vi "HFRR ADV v024 new software.vi"() -> ()   [LabVIEW 2025] (continued)
            n792 = call "IMAGE PATH CREATION PY.vi"("error in (no error)"=w991, "File Name :"=w992) -> ("error out"=w990:errorcluster, "File Path"=w978:path, "File Path String:"=w973:string)  [unwired: 7 in]
            n793 = Match Pattern(string=w986, regular expression=",") -> (before substring=w972:string)  [unwired: 1 in, 3 out]
            n794 = local read "Calibration Tab"() -> (w975:enum32{"Measrument", "Calibrate"})
            n795 = call "Stall Data Flow.vim"("value in"=w990, "milliseconds to wait"=u32 250) -> ("value out"=w974:errorcluster)  [unwired: 1 out]
            n796 = Equal?(x=w972, y="\"rectangle\"") -> (x = y?=w983:bool)
            n797 = case shown="False" w983 {
              tunnel: w982 -> [w1037 w1092]
              tunnel: w979 -> [_ w1083]
              tunnel: cluster{"major":dbl, "minor":dbl, "average":dbl} {"major"=0.0, "minor"=0.0, "average"=0.0} -> [w1035 w1079]
              tunnel: [w1034 w1076] -> w977
              tunnel: w972 -> [w1036 _]
              tunnel: w979 -> [w1033 _]
              frame False {
                n798 = Equal?(x=w1036, y="\"line\"") -> (x = y?=w1038:bool)
                n799 = case shown="True" w1038 {
                  tunnel: w1037 -> [_ w1053]
                  tunnel: w1035 -> [w1040 w1052]
                  tunnel: [w1040 w1050] -> w1034
                  tunnel: w1033 -> [_ w1049]
                  frame False {
                  }
                  frame True {
                    w1048 = 0.0 ("Major Axis")
                    n800 = Match Pattern(string=w1053, regular expression="\"length_px\":") -> (after substring=w1051:string)  [unwired: 1 in, 3 out]
                    n801 = property on="Major Axis" class="DigNum (strict)"("Caption.Text"="") -> ()  [unwired: 2 in, 2 out]
                    n802 = property on="Minor Axis" class="DigNum (strict)"("Caption.Text"="") -> ()  [unwired: 2 in, 2 out]
                    n803 = property on="Average" class="DigNum (strict)"("Caption.Text"="Line") -> ()  [unwired: 2 in, 2 out]
                    n804 = Fract/Exp String To Number(string=w1051, default (0 dbl)=0.0 ("default (0 DBL)")) -> (number=w1047:dbl)  [unwired: 2 in, 1 out]
                    "Pixel Value" <- w1047
                    n805 = Multiply(x=w1047, y=w1049) -> (x*y=w1060:dbl)
                    n806 = Multiply(x=w1060, y=1000.0) -> (x*y=w1043:dbl)
                    n807 = Divide(x=w1043, y=1000.0) -> (x/y=w1046:dbl)
                    n808 = local write "Measurment (mm)"(w1046) -> ()
                    n809 = Bundle By Name(cluster=w1052, "average"=w1043) -> (w1050:cluster{"major":dbl, "minor":dbl, "average":dbl})
                    n810 = Number To Fractional String(number=w1043, precision (6)=i16 1) -> (F-format string=w1042:string)  [unwired: 2 in]
                    n811 = local write "Minor Axis"(w1048) -> ()
                    n812 = local write "Major Axis"(w1048) -> ()
                    n813 = Fract/Exp String To Number(string=w1042) -> (number=w1041:dbl)  [unwired: 3 in, 1 out]
                    n814 = local write "Average"(w1041) -> ()
                  }
                }
              }
              frame True {
                w1080 = 1000.0 ("y")
                w1086 = 0.0 ("default (0 DBL)")
                n815 = Match Pattern(string=w1092, regular expression=" \"width_px\":") -> (after substring=w1090:string)  [unwired: 1 in, 3 out]
                n816 = Match Pattern(string=w1090, regular expression="\"height_px\":") -> (before substring=w1088:string, after substring=w1087:string)  [unwired: 1 in, 2 out]
                n817 = Fract/Exp String To Number(string=w1088, default (0 dbl)=w1086) -> (number=w1085:dbl)  [unwired: 2 in, 1 out]
                n818 = Fract/Exp String To Number(string=w1087, default (0 dbl)=w1086) -> (number=w1084:dbl)  [unwired: 2 in, 1 out]
                n819 = Multiply(x=w1085, y=w1083) -> (x*y=w1082:dbl)
                n820 = Multiply(x=w1084, y=w1083) -> (x*y=w1081:dbl)
                n821 = Multiply(x=w1082, y=w1080) -> (x*y=w1066:dbl)
                n822 = Multiply(x=w1081, y=w1080) -> (x*y=w1064:dbl)
                n823 = Add(x=w1066, y=w1064) -> (x+y=w1078:dbl)
                n824 = property on="Major Axis" class="DigNum (strict)"("Caption.Text"="Major Axis") -> ()  [unwired: 2 in, 2 out]
                n825 = property on="Minor Axis" class="DigNum (strict)"("Caption.Text"="Minor Axis") -> ()  [unwired: 2 in, 2 out]
                n826 = property on="Average" class="DigNum (strict)"("Caption.Text"="Average") -> ()  [unwired: 2 in, 2 out]
                n827 = Divide(x=w1078, y=2.0) -> (x/y=w1062:dbl)
                n828 = Bundle By Name(cluster=w1079, "major"=w1066, "minor"=w1064, "average"=w1062) -> (w1076:cluster{"major":dbl, "minor":dbl, "average":dbl})
                n829 = Number To Fractional String(number=w1064, precision (6)=i16 1) -> (F-format string=w1071:string)  [unwired: 2 in]
                n830 = Number To Fractional String(number=w1062, precision (6)=i16 1) -> (F-format string=w1072:string)  [unwired: 2 in]
                n831 = Number To Fractional String(number=w1066, precision (6)=i16 1) -> (F-format string=w1070:string)  [unwired: 2 in]
                n832 = Fract/Exp String To Number(string=w1071) -> (number=w1063:dbl)  [unwired: 3 in, 1 out]
                n833 = Fract/Exp String To Number(string=w1072) -> (number=w1061:dbl)  [unwired: 3 in, 1 out]
                n834 = Fract/Exp String To Number(string=w1070) -> (number=w1065:dbl)  [unwired: 3 in, 1 out]
                n835 = local write "Major Axis"(w1065) -> ()
                n836 = local write "Average"(w1061) -> ()
                n837 = local write "Minor Axis"(w1063) -> ()
              }
            }
            n838 = case shown="\"Measrument\", Default" w975 {
              tunnel: w978 -> [w1005 _]
              tunnel: w977 -> [w1004 _]
              tunnel: [w1001 w1030] -> w976
              tunnel: w974 -> [w1003 w1030]
              tunnel: w973 -> [w1002 _]
              tunnel: w970 -> [w1000 _]
              frame "Measrument", Default {
                n839 = stacked-sequence {
                  tunnel: w1005 -> [w1023 _]
                  tunnel: w1004 -> [w1021 _]
                  tunnel: w1003 -> [w1019 _]
                  tunnel: w1002 -> [w1018 _]
                  tunnel: [w1013 _] -> w1001
                  tunnel: w1000 -> [w1006 _]
                  frame #0 {
                    n840 = call "IMAGE ANALYSIS.vi"("Enum"=POST_ANALYSIS_ENUM."SAVE IMAGE", "error in"=w1019, "IMAGE FILE PATH"=w1018) -> ("error out"=w1017:errorcluster)  [unwired: 7 in, 1 out]
                    n841 = call "Stall Data Flow.vim"("value in"=w1017, "milliseconds to wait"=u32 1000) -> ("value out"=w1008:errorcluster)  [unwired: 1 out]
                    n842 = local read "Test File List :"() -> (w1025:string)
                    n843 = call "IMAGE ANALYSIS.vi"("Enum"=POST_ANALYSIS_ENUM."MINIMIZE UI", "error in"=w1008) -> ("error out"=w1015:errorcluster)  [unwired: 8 in, 1 out]
                    n844 = Bundle By Name(cluster=T25 {"File Name"="", "Test Method"="", "Operator"="", "Fuel Description"="", "Date and time"=""} ("Main Ref"), "Test Method"=w1006, "File Name"=w1025) -> (w1026:T25)
                    n845 = call "Stall Data Flow.vim"("value in"=w1015, "milliseconds to wait"=u32 1500) -> ("value out"=w1010:errorcluster)  [unwired: 1 out]
                    n846 = call "duf file read.vi"("error in (no error)"=w1010, "Main Ref"=w1026) -> ("error out"=w1024:errorcluster, "Main Ref 2"=w1022:T25)  [unwired: 8 in]
                    n847 = call "DETECTION REPORT for manual.vi"("error in (no error)"=w1024, "return value 3"=w1021, "Image File Path"=w1023, "Main Ref"=w1022) -> ("error out"=w1020:errorcluster)  [unwired: 7 in]
                    n848 = call <vilib>:"Clear Errors.vi"("error in (no error)"=w1020) -> ("error out"=w1011:errorcluster)  [unwired: 5 in, 1 out]
                    n849 = call "IMAGE ANALYSIS.vi"("Enum"=POST_ANALYSIS_ENUM."MINIMIZE UI", "error in"=w1011) -> ("error out"=w1013:errorcluster)  [unwired: 8 in, 1 out]
                  }
                  frame #1 {
                    n850 = local write "Main Tab"(T2."HOME" ("Main Tab")) -> ()
                    n851 = local write "Main Dashboard Buttons"(T1."Home" ("Main Dashboard Buttons")) -> ()
                  }
                }
              }
              frame "Calibrate" {
              }
            }
          }
          frame #2 {
            n852 = Not(x=w1095) -> (.not. x?=w1094:bool)
            n853 = local write "Confirm Measrurement"(w1094) -> ()
            n854 = local read "Calibration Tab"() -> (w1093:enum32{"Measrument", "Calibrate"})
            n855 = case shown="\"Measrument\", Default" w1093 {
              frame "Measrument", Default {
                (unwired) T20."HOME" ("Main Tab")
                n856 = local write "Main Tab"(T2."HOME" ("Main Tab")) -> ()
              }
              frame "Calibrate" {
              }
            }
          }
        }
      }
    }
    n857 = local read "Humidity"() -> (w838:bool)
    n858 = local read "Save Change"() -> (w843:bool)
    n859 = local read "Calibrate"() -> (w844:bool)
    n860 = local read "Auto Start Test"() -> (w839:bool)
    n861 = case shown="True" w844 {
      selector: w844 -> [_ w951]
      frame False {
      }
      frame True {
        n862 = Not(x=w951) -> (.not. x?=w950:bool)
        n863 = local write "Calibrate"(w950) -> ()
        n864 = local write "Calibration Tab"(enum32{"Measrument", "Calibrate"}."Calibrate" ("Calibration Tab")) -> ()
      }
    }
    n865 = case shown="True" w843 {
      selector: w843 -> [_ w895]
      frame False {
      }
      frame True {
        n866 = stacked-sequence {
          tunnel: w895 -> [_ _ _ _ w949]
          frame #0 {
            n867 = call "IMAGE ANALYSIS.vi"("Enum"=POST_ANALYSIS_ENUM."HIDE UI") -> ()  [unwired: 9 in, 2 out]
          }
          frame #1 {
            n868 = local read "100x gain"() -> (w897:dbl)
            n869 = local read "10x Gain"() -> (w898:dbl)
            n870 = local read "5x Gain"() -> (w899:dbl)
            n871 = Number To Fractional String(number=w898, width (-)=i16 4, precision (6)=i16 7) -> (F-format string=w920:string)  [unwired: 1 in]
            n872 = Number To Fractional String(number=0.0, width (-)=i16 4, precision (6)=i16 7) -> (F-format string=w915:string)  [unwired: 1 in]
            n873 = Number To Fractional String(number=w897, width (-)=i16 4, precision (6)=i16 7) -> (F-format string=w903:string)  [unwired: 1 in]
            n874 = Number To Fractional String(number=w899, width (-)=i16 10 ("precision (6)"), precision (6)=i16 7) -> (F-format string=w929:string)  [unwired: 1 in]
            n875 = Concatenate Strings("[CH1]" ("string"), w929, " - 5x Gain" ("string"), "\r") -> (w919:string)
            n876 = Concatenate Strings("[CH2]" ("string"), w920, " - 10x Gain" ("string"), "\r") -> (w918:string)
            n877 = Concatenate Strings("[CH3]" ("string"), w915, " - 20x Gain" ("string"), "\r") -> (w909:string)
            n878 = Concatenate Strings("[CH4]" ("string"), w903, " - 100x Gain" ("string"), "\r") -> (w902:string)
            n879 = String To Path(string="C:\\LAB-IQ\\Image Calibrate v01.dcf") -> (path=w932:path)
            n880 = Concatenate Strings(w919, w918, w909, w902) -> (w917:string)
            n881 = call <vilib>:"Write Characters To File.vi"("append to file? (new file:F)"=FALSE, "character string"=w917, "file path (dialog if empty)"=w932) -> ()  [unwired: 2 in, 1 out]
          }
          frame #2 {
            n882 = String To Path(string="C:\\LAB-IQ\\Image Calibrate v01.dcf") -> (path=w935:path)
            n883 = Open/Create/Replace File ("Open File")(file path (use dialog)=w935) -> (refnum out=w936:refnum<file>)  [unwired: 5 in, 2 out]
            n884 = for {
              N: 4 -> [_]
              tunnel: w936 -> [w942]
              i -> [w938]
              n885 = Read from Text File ("Read File")(file (use dialog)=w942) -> (text=w943:string)  [unwired: 3 in, 3 out]
              n886 = String Subset(string=w943, offset (0)=6, length (rest)=10 ("length (rest)")) -> (substring=w939:string)
              n887 = Fract/Exp String To Number(string=w939) -> (number=w937:dbl)  [unwired: 3 in, 1 out]
              n888 = case shown="3" w938 {
                tunnel: w937 -> [w944 w945 _ w946 _]
                frame 0 {
                  n889 = local write "5x Gain"(w944) -> ()
                }
                frame 1 {
                  n890 = local write "10x Gain"(w945) -> ()
                }
                frame 2 {
                }
                frame 3 {
                  n891 = local write "100x gain"(w946) -> ()
                }
                frame 4, Default {
                }
              }
            }
          }
          frame #3 {
            n892 = call "IMAGE ANALYSIS.vi"("Enum"=POST_ANALYSIS_ENUM."SHOW UI") -> ()  [unwired: 9 in, 2 out]
          }
          frame #4 {
            n893 = Not(x=w949) -> (.not. x?=w948:bool)
            n894 = local write "Save Change"(w948) -> ()
          }
        }
      }
    }
    n895 = case shown="False" w839 {
      tunnel: w838 -> [w865 _]
      frame False {
        n896 = case shown="True" w865 {
          frame False {
          }
          frame True {
            n897 = local read "Set Humidity:"() -> (w869:dbl)
            n898 = local read "Set Humidity:"() -> (w872:dbl)
            n899 = local read "Humidity ( %RH )"() -> (w873:dbl)
            n900 = Subtract(x=w869, y=2.0) -> (x-y=w867:dbl)
            n901 = Add(x=w872, y=2.0) -> (x+y=w868:dbl)
            n902 = In Range and Coerce(upper limit=w868, x=w873, lower limit=w867) -> (In Range?=w866:bool)  [unwired: 1 out]
            n903 = case shown="True" w866 {
              frame False {
              }
              frame True {
                n904 = case shown="True" "Manual Humididty Reached" {
                  selector: "Manual Humididty Reached" -> [_ w876]
                  frame False {
                  }
                  frame True {
                    n905 = Not(x=w876) -> (.not. x?=w875:bool)
                    n906 = local write "Manual Humididty Reached"(w875) -> ()
                    n907 = local read "EVENT LOG"() -> (w878:string)
                    n908 = call "Event Log.vi"("Content"="Target Humidity reached", "EVENT LOG"=w878) -> ("EVENT LOG"=w877:string)  [unwired: 8 in, 1 out]
                    n909 = local write "EVENT LOG"(w877) -> ()
                  }
                }
              }
            }
          }
        }
      }
      frame True {
        n910 = local write "Manual Humididty Reached"(TRUE ("Manual Humididty Reached")) -> ()
      }
    }
    n911 = local read "Cap Live Image"() -> (w859:bool)
    n912 = local read "SCAR MEASURMENT"() -> (w862:enum32{"Auto Scar", "Manual Scar"})
    n913 = Wait (ms)(milliseconds to wait=u32 250) -> ()  [unwired: 1 out]
    n914 = Equal?(x=w862, y=enum32{"Auto Scar", "Manual Scar"}."Manual Scar" ("SCAR MEASURMENT")) -> (x = y?=w860:bool)
    n915 = And(x=w860, y=w859) -> (x .and. y?=w858:bool)
    n916 = case shown="True" w858 {
      selector: w858 -> [_ w1174]
      frame False {
      }
      frame True {
        n917 = stacked-sequence {
          tunnel: [_ _ _ w1189 _] -> _
          tunnel: w1174 -> [_ _ _ _ w1196]
          frame #0 {
            w1175 = 0.0
            n918 = local write "Major Axis"(w1175) -> ()
            n919 = local write "Minor Axis"(w1175) -> ()
            n920 = local write "Average"(w1175) -> ()
          }
          frame #1 {
            n921 = call "CAMERA LIVE FEED FGV.vi"("Enum - Menu"=CAMERA_LIVE_FEED_ENUM."CAMERA MINIMIZE") -> ()  [unwired: 9 in, 2 out]
          }
          frame #2 {
            n922 = local read "FILE 3"() -> (w1183:string)
            n923 = call <vilib>:"Trim Whitespace.vi"("string"="C:\\LAB-IQ\\images\\") -> ("trimmed string"=w1185:string)  [unwired: 1 in]
            n924 = String To Path(string=w1185) -> (path=w1184:path)
            n925 = Concatenate Strings(w1183, ".png" ("string")) -> (w1182:string)
            n926 = Build Path(base path=w1184, name or relative path=w1182) -> (appended path=w1180:path)
            n927 = Path To String(path=w1180) -> (string=w1179:string)
            n928 = call "CAMERA LIVE FEED FGV.vi"("Enum - Menu"=CAMERA_LIVE_FEED_ENUM."CAMERA SAVE", "Image Path"=w1179) -> ("error out"=w1177:errorcluster)  [unwired: 8 in, 1 out]
            n929 = case shown="No Error" w1177 {
              frame No Error {
                n930 = One Button Dialog(message="Image saved successfully") -> ()  [unwired: 1 in, 1 out]
              }
              frame Error {
              }
            }
          }
          frame #3 {
            n931 = call "LIST FILE NAMES.vi"() -> ("error out"=w1191:errorcluster, "filenames"=w1188:string[])  [unwired: 10 in]
            n932 = call "IMAGE ANALYSIS.vi"("Enum"=POST_ANALYSIS_ENUM."SHOW UI", "error in"=w1191) -> ("error out"=w1189:errorcluster)  [unwired: 8 in, 1 out]
            n933 = property on="Test File List :" class="CmbBox"("Strings[]"=w1188) -> ()  [unwired: 2 in, 2 out]
          }
          frame #4 {
            (unwired) T24."Report" ("Main Dashboard Buttons")
            (unwired) T26."Report" ("Main Dashboard Buttons")
            n934 = Not(x=w1196) -> (.not. x?=w1195:bool)
            n935 = local write "Zoom Factore"(0.0 ("Zoom Factore")) -> ()
            n936 = local write "Cap Live Image"(w1195) -> ()
            n937 = local write "Main Tab"(T2."Adv Scar Report" ("Main Tab")) -> ()
            n938 = property on="Cap Live Image" class="Bool (strict)"("BoolText.Text"="Capture Image" ("Boolean Text.Text")) -> ()  [unwired: 2 in, 2 out]
            n939 = local write "Main Dashboard Buttons"(T1."Report" ("Main Dashboard Buttons")) -> ()
          }
        }
      }
    }
    n940 = local read "change Gain"() -> (w842:bool)
    n941 = local read "Back Square"() -> (w841:bool)
    n942 = case shown="True" w842 {
      selector: w842 -> [_ w886]
      frame False {
      }
      frame True {
        n943 = stacked-sequence {
          tunnel: w886 -> [_ w894]
          frame #0 {
            n944 = local read "Actual (µm)"() -> (w890:dbl)
            n945 = local read "Pixel Value"() -> (w889:dbl)
            n946 = local read "Magnification :"() -> (w888:string)
            n947 = Divide(x=w890, y=w889) -> (x/y=w887:dbl)
            n948 = case shown="\"10x\"" w888 {
              tunnel: w887 -> [w891 w892]
              frame "10x" {
                n949 = local write "10x Gain"(w891) -> ()
              }
              frame "5x", Default {
                n950 = local write "5x Gain"(w892) -> ()
              }
            }
          }
          frame #1 {
            n951 = Not(x=w894) -> (.not. x?=w893:bool)
            n952 = local write "change Gain"(w893) -> ()
          }
        }
      }
    }
    n953 = case shown="True" w841 {
      selector: w841 -> [_ w884]
      frame False {
      }
      frame True {
        n954 = Not(x=w884) -> (.not. x?=w883:bool)
        n955 = local write "Back Square"(w883) -> ()
        n956 = local write "Calibration Tab"(enum32{"Measrument", "Calibrate"}."Measrument" ("Calibration Tab")) -> ()
      }
    }
    n957 = local read "Rectangle Tool"() -> (w853:bool)
    n958 = local read "Clear ROI Tool"() -> (w852:bool)
    n959 = local read "Open Image"() -> (w857:bool)
    n960 = local read "line tool"() -> (w854:bool)
    n961 = local read "OUT"() -> (w855:bool)
    n962 = local read "In"() -> (w856:bool)
    n963 = case shown="True" w857 {
      selector: w857 -> [_ w1162]
      tunnel: [w1158 w1164] -> _
      tunnel: w847 -> [w1158 w1163]
      frame False {
      }
      frame True {
        n964 = Not(x=w1162) -> (.not. x?=w1161:bool)
        n965 = local write "Open Image"(w1161) -> ()
        n966 = call "IMAGE ANALYSIS.vi"("Enum"=POST_ANALYSIS_ENUM."HIDE UI", "error in"=w1163) -> ("error out"=w1171:errorcluster)  [unwired: 8 in, 1 out]
        n967 = call "File Dialog"("start path"=path "C:/LAB-IQ/images", "error in"=w1171) -> ("selected path"=w1160:path, "error out"=w1169:errorcluster)  [unwired: 10 in, 2 out]
        "Image path  2" <- w1160
        n968 = call <vilib>:"Clear Errors.vi"("error in (no error)"=w1169) -> ("error out"=w1168:errorcluster)  [unwired: 5 in, 1 out]
        n969 = call "IMAGE ANALYSIS.vi"("Enum"=POST_ANALYSIS_ENUM."OPEN FILE", "error in"=w1168, "File Path"=w1160) -> ("error out"=w1167:errorcluster)  [unwired: 7 in, 1 out]
        n970 = call <vilib>:"Clear Errors.vi"("error in (no error)"=w1167) -> ("error out"=w1166:errorcluster)  [unwired: 5 in, 1 out]
        n971 = call "IMAGE ANALYSIS.vi"("Enum"=POST_ANALYSIS_ENUM."SHOW UI", "error in"=w1166) -> ("error out"=w1164:errorcluster)  [unwired: 8 in, 1 out]
        n972 = local write "Zoom Factore"(100.0 ("Zoom Factore")) -> ()
      }
    }
    n973 = case shown="True" w855 {
      selector: w855 -> [_ w1143]
      tunnel: w847 -> [w1140 w1148]
      tunnel: [w1140 w1142] -> _
      frame False {
      }
      frame True {
        n974 = Not(x=w1143) -> (.not. x?=w1141:bool)
        n975 = local read "Zoom Factore"() -> (w1146:dbl)
        n976 = local write "OUT"(w1141) -> ()
        n977 = call "IMAGE ANALYSIS.vi"("Enum"=POST_ANALYSIS_ENUM."ZOOM OUT", "error in"=w1148) -> ("error out"=w1142:errorcluster)  [unwired: 8 in, 1 out]
        n978 = Divide(x=w1146, y=1.2) -> (x/y=w1144:dbl)
        n979 = local write "Zoom Factore"(w1144) -> ()
      }
    }
    n980 = case shown="True" w856 {
      selector: w856 -> [_ w1152]
      tunnel: w847 -> [w1149 w1157]
      tunnel: [w1149 w1150] -> _
      frame False {
      }
      frame True {
        n981 = Not(x=w1152) -> (.not. x?=w1151:bool)
        n982 = local read "Zoom Factore"() -> (w1155:dbl)
        n983 = local write "In"(w1151) -> ()
        n984 = call "IMAGE ANALYSIS.vi"("Enum"=POST_ANALYSIS_ENUM."ZOOM IN", "error in"=w1157) -> ("error out"=w1150:errorcluster)  [unwired: 8 in, 1 out]
        n985 = Multiply(x=w1155, y=1.2) -> (x*y=w1153:dbl)
        n986 = local write "Zoom Factore"(w1153) -> ()
      }
    }
    n987 = case shown="True" w852 {
      selector: w852 -> [_ w1124]
      tunnel: w847 -> [w1122 w1126]
      tunnel: [w1122 w1125] -> _
      frame False {
      }
      frame True {
        n988 = Not(x=w1124) -> (.not. x?=w1123:bool)
        n989 = local write "Clear ROI Tool"(w1123) -> ()
        n990 = call "IMAGE ANALYSIS.vi"("Enum"=POST_ANALYSIS_ENUM."CLEAR ROI", "error in"=w1126) -> ("error out"=w1125:errorcluster)  [unwired: 8 in, 1 out]
      }
    }
    n991 = case shown="True" w854 {
      selector: w854 -> [_ w1136]
      tunnel: w847 -> [w1134 w1139]
      tunnel: [w1134 w1137] -> _
      frame False {
      }
      frame True {
        n992 = Not(x=w1136) -> (.not. x?=w1135:bool)
        n993 = local write "line tool"(w1135) -> ()
        n994 = call "IMAGE ANALYSIS.vi"("Enum"=POST_ANALYSIS_ENUM."DRAW LINE", "error in"=w1139) -> ("error out"=w1137:errorcluster)  [unwired: 8 in, 1 out]
      }
    }
    n995 = case shown="True" w853 {
      selector: w853 -> [_ w1130]
      tunnel: w847 -> [w1128 w1132]
      tunnel: [w1128 w1131] -> _
      frame False {
      }
      frame True {
        n996 = Not(x=w1130) -> (.not. x?=w1129:bool)
        n997 = local write "Rectangle Tool"(w1129) -> ()
        n998 = call "IMAGE ANALYSIS.vi"("Enum"=POST_ANALYSIS_ENUM."DRAW REC", "error in"=w1132) -> ("error out"=w1131:errorcluster)  [unwired: 8 in, 1 out]
      }
    }
    n999 = local read "SCAR MEASURMENT"() -> (w840:enum32{"Auto Scar", "Manual Scar"})
    n1000 = local read "Fit to Screen Tool"() -> (w849:bool)
    n1001 = local read "Resize Tool"() -> (w848:bool)
    n1002 = case shown="\"Manual Scar\", Default" w840 {
      frame "Auto Scar" {
        n1003 = property on="Cap Live Image" class="Bool (strict)"("BoolText.Text"="Report" ("Boolean Text.Text")) -> ()  [unwired: 2 in, 2 out]
      }
      frame "Manual Scar", Default {
        n1004 = property on="Cap Live Image" class="Bool (strict)"("BoolText.Text"="Save Image" ("Boolean Text.Text")) -> ()  [unwired: 2 in, 2 out]
      }
    }
    n1005 = local read "ROI Color Tool"() -> (w850:bool)
    n1006 = local read "Pan Tool"() -> (w851:bool)
    n1007 = case shown="True" w851 {
      selector: w851 -> [_ w1118]
      tunnel: w847 -> [w1116 w1120]
      tunnel: [w1116 w1119] -> _
      frame False {
      }
      frame True {
        n1008 = Not(x=w1118) -> (.not. x?=w1117:bool)
        n1009 = call "IMAGE ANALYSIS.vi"("Enum"=POST_ANALYSIS_ENUM."PAN", "error in"=w1120) -> ("error out"=w1119:errorcluster)  [unwired: 8 in, 1 out]
        n1010 = local write "Pan Tool"(w1117) -> ()
      }
    }
    n1011 = case shown="True" w848 {
      selector: w848 -> [_ w1102]
      tunnel: w847 -> [w1097 w1099]
      tunnel: [w1097 w1098] -> _
      frame False {
      }
      frame True {
        n1012 = Not(x=w1102) -> (.not. x?=w1101:bool)
        n1013 = local write "Resize Tool"(w1101) -> ()
        n1014 = call "IMAGE ANALYSIS.vi"("Enum"=POST_ANALYSIS_ENUM."RESIZE MODE", "error in"=w1099) -> ("error out"=w1098:errorcluster)  [unwired: 8 in, 1 out]
      }
    }
    n1015 = case shown="True" w849 {
      selector: w849 -> [_ w1107]
      tunnel: [w1103 w1108] -> _
      tunnel: w847 -> [w1103 w1106]
      frame False {
      }
      frame True {
        n1016 = Not(x=w1107) -> (.not. x?=w1105:bool)
        n1017 = local write "Zoom Factore"(100.0 ("Zoom Factore")) -> ()
        n1018 = local write "Fit to Screen Tool"(w1105) -> ()
        n1019 = call "IMAGE ANALYSIS.vi"("Enum"=POST_ANALYSIS_ENUM."FIT", "error in"=w1106) -> ("error out"=w1108:errorcluster)  [unwired: 8 in, 1 out]
      }
    }
    n1020 = case shown="True" w850 {
      selector: w850 -> [_ w1113]
      tunnel: [w1110 w1114] -> _
      tunnel: w847 -> [w1110 w1111]
      frame False {
      }
      frame True {
        n1021 = Not(x=w1113) -> (.not. x?=w1112:bool)
        n1022 = local write "ROI Color Tool"(w1112) -> ()
        n1023 = call "IMAGE ANALYSIS.vi"("Enum"=POST_ANALYSIS_ENUM."SET ROI COLOR", "error in"=w1111) -> ("error out"=w1114:errorcluster)  [unwired: 8 in, 1 out]
      }
    }
    n1024 = local read "Quit"() -> (w864:bool)
  }
  n1025 = while {
    stop <- w1198 stop-if-true
    n1026 = local read "Image Path"() -> (w1201:path)
    n1027 = local read "Print 3"() -> (w1204:bool)
    n1028 = Equal?(x=w1201, y=path "") -> (x = y?=w1200:bool)
    n1029 = Not(x=w1200) -> (.not. x?=w1199:bool)
    n1030 = property on="Print 3" class="Bool (strict)"("Visible"=w1199) -> ()  [unwired: 2 in, 2 out]
    n1031 = case shown="True" w1204 {
      frame False {
        n1032 = local write "Rd"(TRUE ("Boolean 7")) -> ()
      }
      frame True {
        n1033 = flat-sequence {
          tunnel: [w1244] -> w1212
          tunnel: [w1231] -> w1210
          tunnel: [w1241] -> w1206
          tunnel: w1212 -> [w1253]
          tunnel: [w1253] -> w1211
          tunnel: w1210 -> [w1252]
          tunnel: [w1252] -> w1209
          tunnel: [w1250] -> w1208
          tunnel: [w1249] -> w1207
          tunnel: w1206 -> [w1249]
          tunnel: w1211 -> [w1255]
          tunnel: w1209 -> [w1256]
          tunnel: w1208 -> [_]
          tunnel: w1207 -> [w1254]
          frame #0 {
            n1034 = case shown="True" "Rd" {
              frame False {
              }
              frame True {
                n1035 = while {
                  tunnel: "abcdefABCDEF" ("string 2") -> [w1223]
                  shift-right: [w1221] -> w1215
                  shift-left: "" -> [w1220]
                  i -> [w1230]
                  stop <- w1229 stop-if-true
                  n1036 = Random Number (0-1)() -> (number: 0 to 1=w1224:dbl)
                  n1037 = Multiply(x=w1224, y=62.0) -> (x*y=w1226:dbl)
                  n1038 = Decrement(x="Length 2") -> (x-1=w1219:i16)
                  n1039 = To Word Integer(number=w1226) -> (16bit integer=w1227:i16)
                  n1040 = String Subset(string=w1223, offset (0)=w1227, length (rest)=1 ("length (rest)")) -> (substring=w1222:string)
                  n1041 = Greater Or Equal?(x=w1230, y=w1219) -> (x >= y?=w1229:bool)
                  n1042 = Concatenate Strings(w1222, w1220) -> (w1221:string)
                }
                "String 10" <- w1215
                n1043 = local write "Rd"(FALSE ("Boolean 7")) -> ()
              }
            }
          }
          frame #1 {
            w1242 = "_resized.jpg" ("command line")
            (unwired) ".jpg -resize 320x240 " ("string")
            (unwired) "Choose an Image File" ("prompt")
            # "-resize 1798x425"
            n1044 = local read "Image Path"() -> (w1236:path)
            n1045 = Strip Path(path=w1236) -> (stripped path=w1231:path, name=w1232:string)
            n1046 = Match Pattern(string=w1232, regular expression=".jpg") -> (before substring=→"before substring 2":string, after substring=→"after substring":string)  [unwired: 1 in, 2 out]
            n1047 = Match Pattern(string=w1232, regular expression="\\") -> (before substring=w1238:string)  [unwired: 1 in, 3 out]
            n1048 = Match Pattern(string=w1238, regular expression=".jpg") -> (before substring=w1237:string)  [unwired: 1 in, 3 out]
            n1049 = Concatenate Strings("cmd /c convert " ("string"), w1237, ".jpg -resize 320x240  " ("command line"), w1237, w1242) -> (w1245:string)
            n1050 = call <vilib>:"System Exec.vi"("run minimized? (F)"=TRUE, "wait until completion? (T)"=TRUE, "working directory"=w1231, "command line"=w1245) -> ("error out"=w1244:errorcluster)  [unwired: 4 in, 3 out]
            "error out 2" <- w1244
            n1051 = Concatenate Strings(w1237, w1242) -> (w1241:string)
          }
          frame #2 {
            n1052 = Wait (ms)(milliseconds to wait=u32 2000 ("millisecond timer value")) -> (millisecond timer value=w1250:u32)
          }
          frame #3 {
            n1053 = case shown="No Error" w1255 {
              tunnel: w1256 -> [w1259 _]
              tunnel: w1254 -> [w1257 _]
              frame No Error {
                (unwired) ".jpg" ("string")
                n1054 = Path To String(path=w1259) -> (string=w1263:string)
                n1055 = Concatenate Strings(w1263, "\\" ("string"), w1257) -> (w1262:string)
                n1056 = String To Path(string=w1262) -> (path=w1261:path)
                n1057 = call <vilib>:"Read JPEG File.vi"("path to JPEG file"=w1261) -> ("image data"=w1265:T16)  [unwired: 8 in, 2 out]
                "image data" <- w1265
                n1058 = local write "Print 3"(FALSE ("Print 2")) -> ()
                n1059 = call <vilib>:"Draw Flattened Pixmap.vi"("image data"=w1265) -> ("new picture"=→"new picture":picture)  [unwired: 8 in]
              }
              frame Error {
              }
            }
          }
        }
      }
    }
    n1060 = Wait (ms)(milliseconds to wait=u32 20 ("millisecond timer value")) -> ()  [unwired: 1 out]
    n1061 = local read "Quit"() -> (w1198:bool)
  }
  n1062 = while {
    tunnel: w40 -> [_]
    tunnel: w24 -> [_]
    stop <- w1296 stop-if-true
    # "New Adv Logics"
    n1063 = local read "Main Tab"() -> (w1276:T2)
    n1064 = local read "Main Tab"() -> (w1294:T2)
    n1065 = local read "Sign In"() -> (w1293:bool)
    n1066 = case shown="\"Adv Scar\"" w1276 {
      frame "HOME", Default {
        n1067 = local read "LIVE FEED MIN TEMP"() -> (w1429:bool)
        n1068 = local write "LIVE FEED MAX TEMP"(TRUE ("LIVE FEED MAX TEMP")) -> ()
        n1069 = local read "CAMERA ROI MIN TEMP"() -> (w1427:bool)
        n1070 = case shown="True" w1429 {
          selector: w1429 -> [_ w1436]
          frame False {
          }
          frame True {
            n1071 = Not(x=w1436) -> (.not. x?=w1435:bool)
            n1072 = local write "LIVE FEED MIN TEMP"(w1435) -> ()
            n1073 = call "CAMERA LIVE FEED FGV.vi"("Enum - Menu"=CAMERA_LIVE_FEED_ENUM."CAMERA MINIMIZE") -> ()  [unwired: 9 in, 2 out]
          }
        }
        n1074 = case shown="True" w1427 {
          selector: w1427 -> [_ w1433]
          frame False {
          }
          frame True {
            n1075 = Not(x=w1433) -> (.not. x?=w1432:bool)
            n1076 = local write "CAMERA ROI MIN TEMP"(w1432) -> ()
            n1077 = call "IMAGE ANALYSIS.vi"("Enum"=POST_ANALYSIS_ENUM."MINIMIZE UI") -> ()  [unwired: 9 in, 2 out]
          }
        }
        n1078 = local write "CAMERA ROI MAX TEMP"(TRUE ("CAMERA ROI MAX TEMP")) -> ()
      }
      frame "Test Setup" {
        n1079 = local read "LIVE FEED MIN TEMP"() -> (w1439:bool)
        n1080 = local read "CAMERA ROI MIN TEMP"() -> (w1437:bool)
        n1081 = local write "LIVE FEED MAX TEMP"(TRUE ("LIVE FEED MAX TEMP")) -> ()
        n1082 = case shown="True" w1439 {
          selector: w1439 -> [_ w1446]
          frame False {
          }
          frame True {
            n1083 = Not(x=w1446) -> (.not. x?=w1445:bool)
            n1084 = local write "LIVE FEED MIN TEMP"(w1445) -> ()
            n1085 = call "CAMERA LIVE FEED FGV.vi"("Enum - Menu"=CAMERA_LIVE_FEED_ENUM."CAMERA MINIMIZE") -> ()  [unwired: 9 in, 2 out]
          }
        }
        n1086 = case shown="True" w1437 {
          selector: w1437 -> [_ w1443]
          frame False {
          }
          frame True {
            n1087 = Not(x=w1443) -> (.not. x?=w1442:bool)
            n1088 = local write "CAMERA ROI MIN TEMP"(w1442) -> ()
            n1089 = call "IMAGE ANALYSIS.vi"("Enum"=POST_ANALYSIS_ENUM."MINIMIZE UI") -> ()  [unwired: 9 in, 2 out]
          }
        }
        n1090 = local write "CAMERA ROI MAX TEMP"(TRUE ("CAMERA ROI MAX TEMP")) -> ()
      }
      frame "Acquire" {
        n1091 = local read "LIVE FEED MIN TEMP"() -> (w1449:bool)
        n1092 = local write "LIVE FEED MAX TEMP"(TRUE ("LIVE FEED MAX TEMP")) -> ()
        n1093 = local read "CAMERA ROI MIN TEMP"() -> (w1447:bool)
        n1094 = case shown="True" w1449 {
          selector: w1449 -> [_ w1456]
          frame False {
          }
          frame True {
            n1095 = Not(x=w1456) -> (.not. x?=w1455:bool)
            n1096 = local write "LIVE FEED MIN TEMP"(w1455) -> ()
            n1097 = call "CAMERA LIVE FEED FGV.vi"("Enum - Menu"=CAMERA_LIVE_FEED_ENUM."CAMERA MINIMIZE") -> ()  [unwired: 9 in, 2 out]
          }
        }
        n1098 = case shown="True" w1447 {
          selector: w1447 -> [_ w1453]
          frame False {
          }
          frame True {
            n1099 = Not(x=w1453) -> (.not. x?=w1452:bool)
            n1100 = local write "CAMERA ROI MIN TEMP"(w1452) -> ()
            n1101 = call "IMAGE ANALYSIS.vi"("Enum"=POST_ANALYSIS_ENUM."MINIMIZE UI") -> ()  [unwired: 9 in, 2 out]
          }
        }
        n1102 = local write "CAMERA ROI MAX TEMP"(TRUE ("CAMERA ROI MAX TEMP")) -> ()
      }
      frame "Adv Scar" {
        n1103 = local read "CAMERA ROI MIN TEMP"() -> (w1457:bool)
        n1104 = case shown="True" "LIVE FEED MAX TEMP" {
          selector: "LIVE FEED MAX TEMP" -> [_ w1478]
          frame False {
          }
          frame True {
            n1105 = Not(x=w1478) -> (.not. x?=w1477:bool)
            n1106 = local write "LIVE FEED MAX TEMP"(w1477) -> ()
            n1107 = call "CAMERA LIVE FEED FGV.vi"("Enum - Menu"=CAMERA_LIVE_FEED_ENUM."CAMERA RESTORE") -> ("error out"=w1468:errorcluster)  [unwired: 9 in, 1 out]
            n1108 = Type Cast(type=30, x=0) -> (*(type *) &x=w1472:i32)
            n1109 = Add(x=w1472, y=48) -> (x+y=w1473:i32)
            n1110 = call "CAMERA LIVE FEED FGV.vi"("Enum - Menu"=CAMERA_LIVE_FEED_ENUM."CAMERA MODE SET", "error in (no error)"=w1468, "CAMERA MODE"=w1473) -> ("error out"=w1465:errorcluster)  [unwired: 7 in, 1 out]
            n1111 = call "CAMERA LIVE FEED FGV.vi"("Enum - Menu"=CAMERA_LIVE_FEED_ENUM."CAMERA GRAY", "error in (no error)"=w1465) -> ("error out"=w1464:errorcluster)  [unwired: 8 in, 1 out]
            n1112 = call "LIST FILE NAMES.vi"("error in (no error)"=w1464) -> ("error out"=w1474:errorcluster, "filenames"=w1475:string[])  [unwired: 9 in]
            n1113 = property on="FILE 3" class="CmbBox"(error in=w1474, "Strings[]"=w1475) -> ()  [unwired: 1 in, 2 out]
          }
        }
        n1114 = case shown="True" w1457 {
          selector: w1457 -> [_ w1463]
          frame False {
          }
          frame True {
            n1115 = Not(x=w1463) -> (.not. x?=w1462:bool)
            n1116 = local write "CAMERA ROI MIN TEMP"(w1462) -> ()
            n1117 = call "IMAGE ANALYSIS.vi"("Enum"=POST_ANALYSIS_ENUM."MINIMIZE UI") -> ()  [unwired: 9 in, 2 out]
          }
        }
        n1118 = local write "CAMERA ROI MAX TEMP"(TRUE ("CAMERA ROI MAX TEMP")) -> ()
        "LIVE FEED MIN TEMP" <- TRUE ("LIVE FEED MIN TEMP")
      }
      frame "Adv Scar Report" {
        n1119 = local read "CAMERA ROI MAX TEMP"() -> (w1479:bool)
        n1120 = local read "LIVE FEED MIN TEMP"() -> (w1481:bool)
        n1121 = local write "LIVE FEED MAX TEMP"(TRUE ("LIVE FEED MAX TEMP")) -> ()
        n1122 = case shown="True" w1481 {
          selector: w1481 -> [_ w1490]
          frame False {
          }
          frame True {
            n1123 = Not(x=w1490) -> (.not. x?=w1489:bool)
            n1124 = local write "LIVE FEED MIN TEMP"(w1489) -> ()
            n1125 = call "CAMERA LIVE FEED FGV.vi"("Enum - Menu"=CAMERA_LIVE_FEED_ENUM."CAMERA MINIMIZE") -> ()  [unwired: 9 in, 2 out]
          }
        }
        n1126 = case shown="True" w1479 {
          selector: w1479 -> [_ w1487]
          frame False {
          }
          frame True {
            n1127 = Not(x=w1487) -> (.not. x?=w1485:bool)
            n1128 = local write "CAMERA ROI MAX TEMP"(w1485) -> ()
            n1129 = call "IMAGE ANALYSIS.vi"("Enum"=POST_ANALYSIS_ENUM."SHOW UI") -> ("error out"=w1484:errorcluster)  [unwired: 9 in, 1 out]
            n1130 = call "LIST FILE NAMES.vi"("error in (no error)"=w1484) -> ("filenames"=w1483:string[])  [unwired: 9 in, 1 out]
            n1131 = property on="Test File List :" class="CmbBox"("Strings[]"=w1483) -> ()  [unwired: 2 in, 2 out]
          }
        }
        n1132 = local write "CAMERA ROI MIN TEMP"(TRUE ("CAMERA ROI MIN TEMP")) -> ()
      }
      frame "Compare Files" {
        n1133 = local read "LIVE FEED MIN TEMP"() -> (w1493:bool)
        n1134 = local write "LIVE FEED MAX TEMP"(TRUE ("LIVE FEED MAX TEMP")) -> ()
        n1135 = local read "CAMERA ROI MIN TEMP"() -> (w1491:bool)
        n1136 = case shown="True" w1493 {
          selector: w1493 -> [_ w1500]
          frame False {
          }
          frame True {
            n1137 = Not(x=w1500) -> (.not. x?=w1499:bool)
            n1138 = local write "LIVE FEED MIN TEMP"(w1499) -> ()
            n1139 = call "CAMERA LIVE FEED FGV.vi"("Enum - Menu"=CAMERA_LIVE_FEED_ENUM."CAMERA MINIMIZE") -> ()  [unwired: 9 in, 2 out]
          }
        }
        n1140 = case shown="True" w1491 {
          selector: w1491 -> [_ w1497]
          frame False {
          }
          frame True {
            n1141 = Not(x=w1497) -> (.not. x?=w1496:bool)
            n1142 = local write "CAMERA ROI MIN TEMP"(w1496) -> ()
            n1143 = call "IMAGE ANALYSIS.vi"("Enum"=POST_ANALYSIS_ENUM."MINIMIZE UI") -> ()  [unwired: 9 in, 2 out]
          }
        }
        n1144 = local write "CAMERA ROI MAX TEMP"(TRUE ("CAMERA ROI MAX TEMP")) -> ()
      }
      frame "About" {
        n1145 = local read "LIVE FEED MIN TEMP"() -> (w1503:bool)
        n1146 = local write "LIVE FEED MAX TEMP"(TRUE ("LIVE FEED MAX TEMP")) -> ()
        n1147 = local read "CAMERA ROI MIN TEMP"() -> (w1502:bool)
        n1148 = case shown="True" w1503 {
          selector: w1503 -> [_ w1510]
          frame False {
          }
          frame True {
            n1149 = Not(x=w1510) -> (.not. x?=w1509:bool)
            n1150 = local write "LIVE FEED MIN TEMP"(w1509) -> ()
            n1151 = call "CAMERA LIVE FEED FGV.vi"("Enum - Menu"=CAMERA_LIVE_FEED_ENUM."CAMERA MINIMIZE") -> ()  [unwired: 9 in, 2 out]
          }
        }
        n1152 = case shown="True" w1502 {
          selector: w1502 -> [_ w1507]
          frame False {
          }
          frame True {
            n1153 = Not(x=w1507) -> (.not. x?=w1506:bool)
            n1154 = local write "CAMERA ROI MIN TEMP"(w1506) -> ()
            n1155 = call "IMAGE ANALYSIS.vi"("Enum"=POST_ANALYSIS_ENUM."MINIMIZE UI") -> ()  [unwired: 9 in, 2 out]
          }
        }
        n1156 = local write "CAMERA ROI MAX TEMP"(TRUE ("CAMERA ROI MIN TEMP")) -> ()
      }
      frame "Advance" {
        n1157 = local read "LIVE FEED MIN TEMP"() -> (w1513:bool)
        n1158 = local write "LIVE FEED MAX TEMP"(TRUE ("LIVE FEED MAX TEMP")) -> ()
        n1159 = local read "CAMERA ROI MIN TEMP"() -> (w1511:bool)
        n1160 = case shown="True" w1513 {
          selector: w1513 -> [_ w1520]
          frame False {
          }
          frame True {
            n1161 = Not(x=w1520) -> (.not. x?=w1519:bool)
            n1162 = local write "LIVE FEED MIN TEMP"(w1519) -> ()
            n1163 = call "CAMERA LIVE FEED FGV.vi"("Enum - Menu"=CAMERA_LIVE_FEED_ENUM."CAMERA MINIMIZE") -> ()  [unwired: 9 in, 2 out]
          }
        }
        n1164 = local write "CAMERA ROI MAX TEMP"(TRUE ("CAMERA ROI MAX TEMP")) -> ()
        n1165 = case shown="True" w1511 {
          selector: w1511 -> [_ w1517]
          frame False {
          }
          frame True {
            n1166 = Not(x=w1517) -> (.not. x?=w1516:bool)
            n1167 = local write "CAMERA ROI MIN TEMP"(w1516) -> ()
            n1168 = call "IMAGE ANALYSIS.vi"("Enum"=POST_ANALYSIS_ENUM."MINIMIZE UI") -> ()  [unwired: 9 in, 2 out]
          }
        }
      }
      frame "Mooha" {
        n1169 = local read "LIVE FEED MIN TEMP"() -> (w1523:bool)
        n1170 = local write "LIVE FEED MAX TEMP"(TRUE ("LIVE FEED MAX TEMP")) -> ()
        n1171 = local read "CAMERA ROI MIN TEMP"() -> (w1521:bool)
        n1172 = case shown="True" w1523 {
          selector: w1523 -> [_ w1530]
          frame False {
          }
          frame True {
            n1173 = Not(x=w1530) -> (.not. x?=w1529:bool)
            n1174 = local write "LIVE FEED MIN TEMP"(w1529) -> ()
            n1175 = call "CAMERA LIVE FEED FGV.vi"("Enum - Menu"=CAMERA_LIVE_FEED_ENUM."CAMERA MINIMIZE") -> ()  [unwired: 9 in, 2 out]
          }
        }
        n1176 = local write "CAMERA ROI MAX TEMP"(TRUE ("CAMERA ROI MAX TEMP")) -> ()
        n1177 = case shown="True" w1521 {
          selector: w1521 -> [_ w1527]
          frame False {
          }
          frame True {
            n1178 = Not(x=w1527) -> (.not. x?=w1526:bool)
            n1179 = local write "CAMERA ROI MIN TEMP"(w1526) -> ()
            n1180 = call "IMAGE ANALYSIS.vi"("Enum"=POST_ANALYSIS_ENUM."MINIMIZE UI") -> ()  [unwired: 9 in, 2 out]
          }
        }
      }
    }
    n1181 = local read "Auto Start Test"() -> (w1267:bool)
    n1182 = case shown="True" "sign in temp" {
      frame False {
      }
      frame True {
        w1303 = 1 ("y")
        n1183 = local read "USERNAME"() -> (w1309:string)
        n1184 = local read "USER ID"() -> (w1306:string)
        n1185 = call <vilib>:"Trim Whitespace.vi"("string"=w1309) -> ("trimmed string"=w1308:string)  [unwired: 1 in]
        n1186 = call <vilib>:"Trim Whitespace.vi"("string"=w1306) -> ("trimmed string"=w1307:string)  [unwired: 1 in]
        n1187 = String Length(string=w1308) -> (length=w1305:i32)
        n1188 = String Length(string=w1307) -> (length=w1304:i32)
        n1189 = Greater?(x=w1305, y=w1303) -> (0:w1302:bool)
        n1190 = Greater?(x=w1304, y=w1303) -> (0:w1301:bool)
        n1191 = And(x=w1302, y=w1301) -> (x .and. y?=w1300:bool)
        n1192 = case shown="True" w1300 {
          frame False {
            n1193 = property on="Sign In" class="Bool (strict)"("DisabledEnum"=T19."Disabled" ("Disabled")) -> ()  [unwired: 2 in, 2 out]
          }
          frame True {
            n1194 = property on="Sign In" class="Bool (strict)"("DisabledEnum"=T19."Enabled" ("Disabled")) -> ()  [unwired: 2 in, 2 out]
          }
        }
      }
    }
    n1195 = local read "Air Temperature"() -> (w1284:bool)
    n1196 = local read "Coefficient Of Friction"() -> (w1285:bool)
    n1197 = case shown="False" w1267 {
      frame False {
        n1198 = local read "Auto stop temp"() -> (w1297:bool)
        n1199 = case shown="True" w1297 {
          frame False {
          }
          frame True {
            n1200 = local write "Auto Start Temp"(FALSE ("Auto Start Temp")) -> ()
          }
        }
      }
      frame True {
        "Auto stop temp" <- TRUE ("Auto stop temp")
      }
    }
    n1201 = local read "Humidity"() -> (w1283:bool)
    n1202 = case shown="\"HOME\"" w1294 {
      frame "HOME" {
        n1203 = local write "main tab sub"(enum32{"Page 1", "Page 2"}."Page 1" ("main tab sub")) -> ()
      }
      frame Default {
        n1204 = local write "main tab sub"(enum32{"Page 1", "Page 2"}."Page 2" ("main tab sub")) -> ()
      }
    }
    n1205 = case shown="True" w1293 {
      selector: w1293 -> [_ w1644]
      frame False {
      }
      frame True {
        n1206 = Not(x=w1644) -> (.not. x?=w1643:bool)
        n1207 = local write "Sign In"(w1643) -> ()
        n1208 = local write "Main Dashboard Buttons"(T24."Test Setup" ("Main Dashboard Buttons")) -> ()
      }
    }
    n1209 = case shown="\"Numeric Display\", Default" "Num/Graph" {
      frame "Numeric Display", Default {
        n1210 = property on="Single/Multiple" class="RadioBtnsControl (strict)"("Visible"=FALSE) -> ()  [unwired: 2 in, 2 out]
        n1211 = property on="Single - Graph" class="Ring (strict)"("Visible"=FALSE) -> ()  [unwired: 2 in, 2 out]
        n1212 = local write "Main Tab Display"(T4."Dashboard 1" ("Main Tab Display")) -> ()
      }
      frame "Graph Display" {
        n1213 = property on="Single/Multiple" class="RadioBtnsControl (strict)"("Visible"=TRUE) -> ()  [unwired: 2 in, 2 out]
        n1214 = case shown="\"Multiple\"" "Single/Multiple" {
          frame "Single ", Default {
            n1215 = property on="Single - Graph" class="Ring (strict)"("Visible"=TRUE) -> ()  [unwired: 2 in, 2 out]
            n1216 = local write "Main Tab Display"(T4."Dashboard 3" ("Main Tab Display")) -> ()
          }
          frame "Multiple" {
            n1217 = property on="Single - Graph" class="Ring (strict)"("Visible"=FALSE) -> ()  [unwired: 2 in, 2 out]
            n1218 = local write "Main Tab Display"(T4."Dashboard 2" ("Main Tab Display")) -> ()
          }
        }
      }
    }
    n1219 = local read "Stroke"() -> (w1282:bool)
    n1220 = local read "USERNAME"() -> (w1288:string)
    n1221 = local read "USER ID"() -> (w1287:string)
    n1222 = case shown="True" w1285 {
      selector: w1285 -> [_ w1570]
      frame False {
      }
      frame True {
        n1223 = Not(x=w1570) -> (.not. x?=w1569:bool)
        n1224 = local write "Coefficient Of Friction"(w1569) -> ()
        n1225 = local write "Tab Control 2"(T6."Coefficient Of Friction" ("Tab Control 2")) -> ()
      }
    }
    n1226 = case shown="True" w1284 {
      selector: w1284 -> [_ w1567]
      frame False {
      }
      frame True {
        n1227 = Not(x=w1567) -> (.not. x?=w1565:bool)
        n1228 = local write "Air Temperature"(w1565) -> ()
        n1229 = local write "Tab Control 2"(T6."Air Temperature" ("Tab Control 2")) -> ()
      }
    }
    n1230 = local write "Operator ID"(w1287) -> ()
    n1231 = case shown="True" w1282 {
      selector: w1282 -> [_ w1561]
      frame False {
      }
      frame True {
        n1232 = Not(x=w1561) -> (.not. x?=w1559:bool)
        n1233 = local write "Stroke"(w1559) -> ()
        n1234 = local write "Tab Control 2"(T6."Stroke" ("Tab Control 2")) -> ()
      }
    }
    n1235 = local write "tested by"(w1288) -> ()
    n1236 = case shown="True" w1283 {
      selector: w1283 -> [_ w1564]
      frame False {
      }
      frame True {
        n1237 = Not(x=w1564) -> (.not. x?=w1562:bool)
        n1238 = local write "Humidity"(w1562) -> ()
        n1239 = local write "Tab Control 2"(T6."Humidity" ("Tab Control 2")) -> ()
      }
    }
    n1240 = case shown="\"Calibration\"" "Main Dashboard Buttons" {
      tunnel: [T2."HOME" ("Main Tab") T2."Test Setup" ("Main Tab") T2."Acquire" ("Main Tab") T2."Adv Scar" ("Main Tab") T2."Adv Scar Report" ("Main Tab") T2."Compare Files" ("Main Tab") T2."Calibration" ("Main Tab") T2."About" ("Main Tab") T2."Advance" ("Main Tab")] -> w1266
      frame "Home", Default {
      }
      frame "Test Setup" {
      }
      frame "Dashboard" {
      }
      frame "Imaging" {
      }
      frame "Report" {
      }
      frame "Analysis" {
      }
      frame "Calibration" {
      }
      frame "About" {
      }
      frame "Advance" {
      }
    }
    n1241 = Wait (ms)(milliseconds to wait=u32 100) -> ()  [unwired: 1 out]
    n1242 = local read "Main Tab Display"() -> (w1286:T4)
    n1243 = local write "Main Tab"(w1266) -> ()
    n1244 = case shown="\"Dashboard 3\"" w1286 {
      frame "Dashboard 1", Default {
        n1245 = property on="Reset Graph" class="Bool (strict)"("Visible"=FALSE) -> ()  [unwired: 2 in, 2 out]
      }
      frame "Dashboard 2" {
        n1246 = property on="Reset Graph" class="Bool (strict)"("Visible"=TRUE) -> ()  [unwired: 2 in, 2 out]
      }
      frame "Dashboard 3" {
        n1247 = property on="Reset Graph" class="Bool (strict)"("Visible"=TRUE) -> ()  [unwired: 2 in, 2 out]
      }
    }
    n1248 = local read "SCAR MEASURMENT"() -> (w1274:enum32{"Auto Scar", "Manual Scar"})
    n1249 = local read "Humidity"() -> (w1289:bool)
    n1250 = local read "Cap Live Image"() -> (w1271:bool)
    n1251 = local read "Sample Temperature"() -> (w1281:bool)
    n1252 = local read "Air Temp vs Humidity"() -> (w1279:bool)
    n1253 = local read "Frequency"() -> (w1280:bool)
    n1254 = case shown="True" w1289 {
      frame False {
        n1255 = local write "Humidity On Command"(TRUE ("Humidity On Command")) -> ()
        n1256 = case shown="True" "Humidity Off Command" {
          selector: "Humidity Off Command" -> [_ w1577]
          frame False {
          }
          frame True {
            n1257 = stacked-sequence {
              frame #0 {
                n1258 = local read "Write UNO"() -> (w1579:string[])
                n1259 = Insert Into Array(array=w1579, new element="R;1" ("new element/subarray")) -> (w1578:string[])  [unwired: 1 in]
                n1260 = local write "Write UNO"(w1578) -> ()
              }
              frame #1 {
                n1261 = Wait (ms)(milliseconds to wait=u32 2000) -> ()  [unwired: 1 out]
              }
              frame #2 {
                n1262 = local read "Write UNO"() -> (w1582:string[])
                n1263 = local read "EVENT LOG"() -> (w1586:string)
                n1264 = call "Event Log.vi"("Content"="Humidity Control Off" ("string"), "EVENT LOG"=w1586) -> ("EVENT LOG"=w1587:string)  [unwired: 8 in, 1 out]
                n1265 = local write "EVENT LOG"(w1587) -> ()
                n1266 = Insert Into Array(array=w1582, new element="R;1" ("new element/subarray")) -> (w1583:string[])  [unwired: 1 in]
                n1267 = local write "Write UNO"(w1583) -> ()
              }
            }
            n1268 = Not(x=w1577) -> (.not. x?=w1576:bool)
            n1269 = local write "Humidity Off Command"(w1576) -> ()
          }
        }
      }
      frame True {
        n1270 = local write "Humidity Off Command"(TRUE ("Humidity Off Command")) -> ()
        n1271 = case shown="True" "Humidity On Command" {
          selector: "Humidity On Command" -> [_ w1591]
          frame False {
          }
          frame True {
            n1272 = stacked-sequence {
              frame #0 {
                n1273 = local read "Set Rh"() -> (w1597:dbl)
                n1274 = local read "Write UNO"() -> (w1592:string[])
                n1275 = Number To Fractional String(number=w1597, precision (6)=i16 2) -> (F-format string=w1598:string)  [unwired: 2 in]
                n1276 = Concatenate Strings("M;" ("new element/subarray"), w1598) -> (w1596:string)
                n1277 = Insert Into Array(array=w1592, new element=w1596) -> (w1593:string[])  [unwired: 1 in]
                n1278 = local write "Write UNO"(w1593) -> ()
              }
              frame #1 {
                n1279 = Wait (ms)(milliseconds to wait=u32 2000) -> ()  [unwired: 1 out]
              }
              frame #2 {
                n1280 = local read "Set Rh"() -> (w1605:dbl)
                n1281 = local read "Write UNO"() -> (w1600:string[])
                n1282 = Number To Fractional String(number=w1605, precision (6)=i16 2) -> (F-format string=w1606:string)  [unwired: 2 in]
                n1283 = Concatenate Strings("M;" ("new element/subarray"), w1606) -> (w1604:string)
                n1284 = Insert Into Array(array=w1600, new element=w1604) -> (w1601:string[])  [unwired: 1 in]
                n1285 = local write "Write UNO"(w1601) -> ()
              }
              frame #3 {
                n1286 = Wait (ms)(milliseconds to wait=u32 1500) -> ()  [unwired: 1 out]
              }
              frame #4 {
                (unwired) "% RH" ("string")
                (unwired) i16 2 ("precision (6)")
                (unwired) "M;" ("new element/subarray")
                n1287 = local read "Set Rh"() -> (w1615:dbl)
                n1288 = local read "Write UNO"() -> (w1608:string[])
                n1289 = Number To Fractional String(number=w1615, precision (6)=i16 2) -> (F-format string=w1612:string)  [unwired: 2 in]
                n1290 = Concatenate Strings("M;" ("new element/subarray"), w1612) -> (w1616:string)
                n1291 = Concatenate Strings("Humidity Set to : " ("string"), w1612, "% RH" ("string")) -> (w1610:string)
                n1292 = Insert Into Array(array=w1608, new element=w1616) -> (w1609:string[])  [unwired: 1 in]
                n1293 = disable-structure shown="Enabled" {
                  frame Enabled {
                    n1294 = local read "EVENT LOG"() -> (w1619:string)
                    n1295 = call "Event Log.vi"("Content"="Humidity Control On", "EVENT LOG"=w1619) -> ("EVENT LOG"=w1620:string)  [unwired: 8 in, 1 out]
                    n1296 = local write "EVENT LOG"(w1620) -> ()
                  }
                  frame Disabled {
                  }
                }
                n1297 = disable-structure shown="Enabled" {
                  disable-tunnel: w1610 -> [_ _]
                  frame Enabled {
                    n1298 = local read "EVENT LOG"() -> (w1622:string)
                    n1299 = call "Event Log.vi"("Content"="Humidity Control On", "EVENT LOG"=w1622) -> ("EVENT LOG"=w1623:string)  [unwired: 8 in, 1 out]
                    n1300 = local write "EVENT LOG"(w1623) -> ()
                  }
                  frame Disabled {
                  }
                }
                n1301 = local write "Write UNO"(w1609) -> ()
              }
            }
            n1302 = Not(x=w1591) -> (.not. x?=w1590:bool)
            n1303 = local write "Humidity On Command"(w1590) -> ()
          }
        }
      }
    }
    n1304 = Equal?(x=w1274, y=enum32{"Auto Scar", "Manual Scar"}."Auto Scar" ("SCAR MEASURMENT")) -> (x = y?=w1270:bool)
    n1305 = local read "TEST STANDARD"() -> (w1277:T3)
    n1306 = And(x=w1271, y=w1270) -> (x .and. y?=w1272:bool)
    n1307 = case shown="True" w1272 {
      selector: w1272 -> [_ w1376]
      tunnel: errorcluster {"status"=FALSE, "code"=0, "source"=""} ("error in (no error) 3") -> [_ w1377]
      frame False {
      }
      frame True {
        n1308 = stacked-sequence {
          tunnel: w1377 -> [_ _ _ _ _ _ _ w1425]
          tunnel: w1376 -> [_ _ _ _ _ w1406 _ _]
          frame #0 {
